vi "run.vi"(8 "error in (no error)":errorcluster, 11 "GenericScanHead in":refnum<class "GenericScanHead.lvclass">) -> (0 "error out":errorcluster, 3 "GenericScanHead out":refnum<class "GenericScanHead.lvclass">)   [LabVIEW 2010, in "GenericScanHead.lvclass"]
uses:
  GenericScanHead.lvclass
  common/classes/ErrorController/ErrorController/class_data.vi
  common/classes/ErrorController/ErrorController/ErrorController.lvclass
panel:
  # "Functionality not available..."
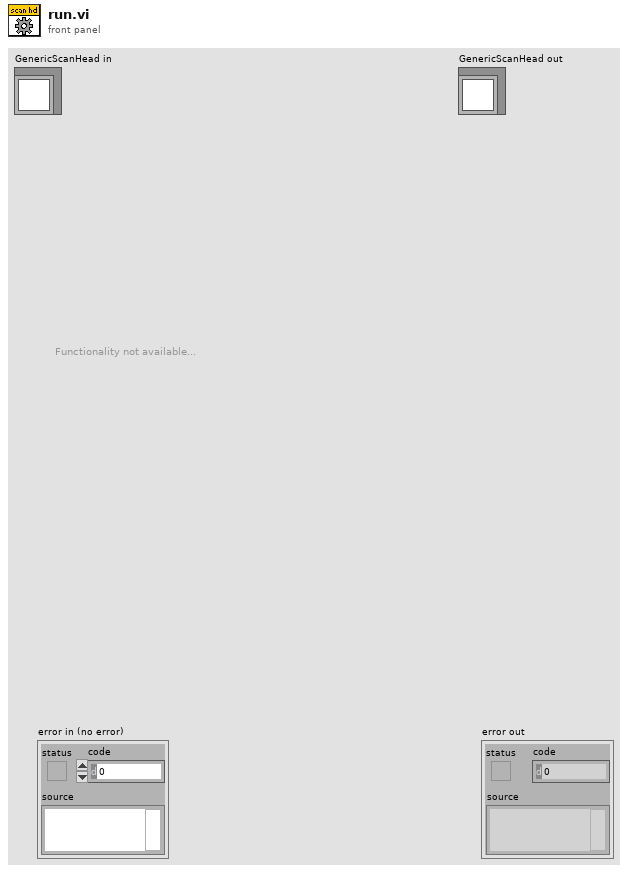
[diagram p1: front panel]
types:
  T1 = typedef "main_trigger_enum.ctl" = enum16{"NULL", "initialise", "terminate", "start", "stop", "change objective", "change experimentController", "change imagingMode", "save notebook", "started saving", "finished saving", "expCtr ready", "expCtr missing", "imgMd ready", "imgMd missing", "scanHd ready", "scanHd missing", "DAQ ready", "DAQ missing", "imgAsm ready", "imgAsm missing", "dataColl ready", "dataColl missing", "display ready", "display missing", "analysr ready", "analysr missing", "instrmnt ready", "instrmnt missing", "stimltr ready", "stimltr missing", "stage ready", "stage missing"}
  T2 = typedef "GenericToplevelComponent.lvclass/common_trigger_enum.ctl" = enum16{"NULL", "initialise", "terminate", "fetch command", "fetch data", "attach observer", "register as observer", "detach observer", "acknowledge", "start", "stop", "sweep started", "sweep finished", "experiment started", "experiment stopped"}
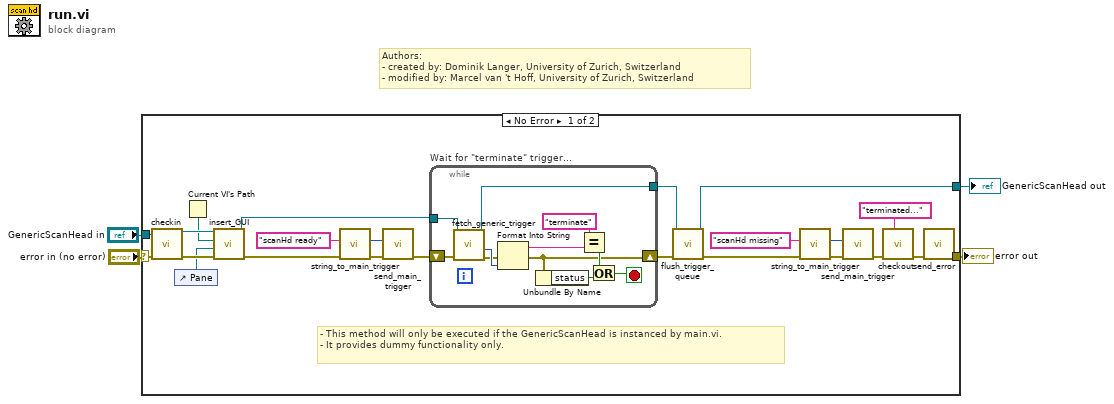
[diagram p0: block diagram]
diagram:
  # "Authors: \n- created by: Dominik Langer, University of Zurich, Switzerland\n- modified by: Marcel van 't Hoff, University of Zurich, Switzerland"
  n1 = case shown="No Error" "error in (no error)" {
    selector: "error in (no error)" -> [w27 w40]
    tunnel: [w19 w40] -> w3
    tunnel: [w15 w39] -> w1
    tunnel: "GenericScanHead in" -> [w26 w39]
    frame No Error {
      # "- This method will only be executed if the GenericScanHead is instanced by main.vi.\n- It provides dummy functionality only."
      n2 = call-dynamic "checkin.vi"("error in (no error)"=w27, "GenericScanHead in"=w26) -> ("error out"=w23:errorcluster, "GenericScanHead out"=w24:refnum<class "GenericScanHead.lvclass">)  [unwired: 8 in]
      n3 = control-ref of="Pane"() -> (w21:refnum<vi>)
      n4 = Current VI's Path() -> (path=w22:path)
      n5 = call-dynamic "insert_GUI.vi"("error in (no error)"=w23, "Pane"=w21, "VI path"=w22, "GenericComponent in"=w24) -> ("error out"=w13:errorcluster, "GenericComponent out"=w17:refnum<class "GenericScanHead.lvclass">)  [unwired: 6 in]
      n6 = call "string_to_main_trigger.vi"("error in (no error)"=w13, "trigger string"="scanHd ready") -> ("error out"=w12:errorcluster, "main trigger"=w10:T1)  [unwired: 8 in]
      n7 = call "send_main_trigger.vi"("error in (no error)"=w12, "trigger"=w10) -> ("error out"=w25:errorcluster)  [unwired: 9 in]
      n8 = while "Wait for \"terminate\" trigger..." {
        shift-right: [w30] -> w18
        shift-left: w25 -> [w38]
        tunnel: w17 -> [w37]
        tunnel: [w36] -> w16
        stop <- w33 stop-if-true
        n9 = call-dynamic "fetch_generic_trigger.vi"("error in (no error)"=w38, "GenericToplevelComponent in"=w37) -> ("error out"=w31:errorcluster, "common trigger"=w32:T2, "GenericToplevelComponent out"=w36:refnum<class "GenericScanHead.lvclass">)  [unwired: 3 in, 4 out]
        n10 = Format Into String(error in=w31, w32) -> (resulting string=w29:string, error out=w30:errorcluster)  [unwired: 2 in]
        n11 = Unbundle By Name(w30) -> ("status"=w35:bool)
        n12 = Equal?(x="terminate", y=w29) -> (x = y?=w34:bool)
        n13 = Or(x=w34, y=w35) -> (x .or. y?=w33:bool)
      }
      n14 = call-dynamic "flush_trigger_queue.vi"("error in (no error)"=w18, "GenericToplevelComponent in"=w16) -> ("error out"=w6:errorcluster, "GenericToplevelComponent out"=w15:refnum<class "GenericScanHead.lvclass">)  [unwired: 8 in]
      n15 = call "string_to_main_trigger.vi"("error in (no error)"=w6, "trigger string"="scanHd missing") -> ("error out"=w7:errorcluster, "main trigger"=w9:T1)  [unwired: 8 in]
      n16 = call "send_main_trigger.vi"("error in (no error)"=w7, "trigger"=w9) -> ("error out"=w5:errorcluster)  [unwired: 9 in]
      n17 = call "checkout.vi"("locked by?"="terminated...", "error in (no error)"=w5) -> ("error out"=w20:errorcluster)  [unwired: 8 in, 1 out]
      n18 = call "send_error.vi"("error in (no error)"=w20) -> ("error out"=w19:errorcluster)  [unwired: 10 in]
    }
    frame Error {
    }
  }
  "error out" <- w3
  "GenericScanHead out" <- w1
